vi "Release.vi"(8 "Error In":errorcluster, 11 "Float In":refnum<class "Float.lvclass">) -> (0 "Error Out":errorcluster)   [LabVIEW 2016, in "Float.lvclass"]
uses:
  Float.lvclass
  Tree Data/Tree Data.lvclass
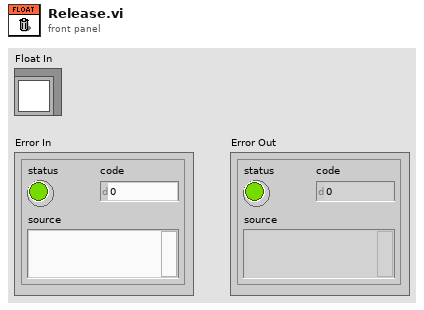
[diagram p1: front panel]
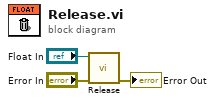
[diagram p0: block diagram]
diagram:
  n1 = call-parent "Release.vi"("Error In"="Error In", "Tree Data In"="Float In") -> ("Error Out"=→"Error Out":errorcluster)  [unwired: 9 in]
